vi "Real Kronecker Product.vi"(10 "B":T1, 11 "A":T1) -> (0 "error":i32, 3 "Kronecker Product":T1)   [LabVIEW 2017, in "NI_AALPro.lvlib"]
doc: "Calculates the Kronecker product of the input matrices <B>A</B> and <B>B</B>. The data types you wire to the <B>A</B> and <B>B</B> inputs determine the polymorphic instance to use."
uses:
  NI_AALPro.lvlib
  RealMatrix.ctl
  lvanlys.dll
  NI_Matrix.lvlib
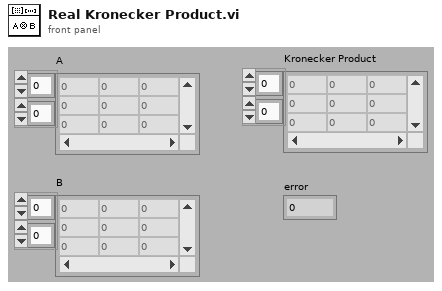
[diagram p1: front panel]
types:
  T1 = typedef "NI_Matrix.lvlib/RealMatrix.ctl" = dbl[][]
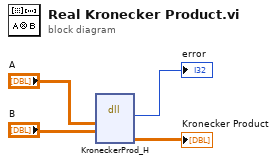
[diagram p0: block diagram]
diagram:
  n1 = dll-call lib="C:/Program Files/National Instruments/LabVIEW 2017/resource/lvanlys.*" fn="KroneckerProd_H"("A"="A", "B"="B") -> (→"error":i32, "C"=→"Kronecker Product":dbl[][])  [unwired: 6 in, 2 out]
